vi "EuniceF_Project5.vi"() -> ()   [LabVIEW 2025]
panel:
  out "TemperatureChart":dbl(graph)
  out "RTD":dbl(slide) scale=100.0..110.0
  out "Vp,mV":dbl(slide) scale=0.0..100.0
  out "Vdiff,mV":dbl(slide) scale=0.0..100.0
  out "COLD":bool
  in  "STOP":bool
  out "HOT":bool
  out "Thermometer":dbl(slide) scale=0.0..100.0
  out "Vscc,V":dbl(slide) scale=-10.0..10.0
  out "AtoD":i16
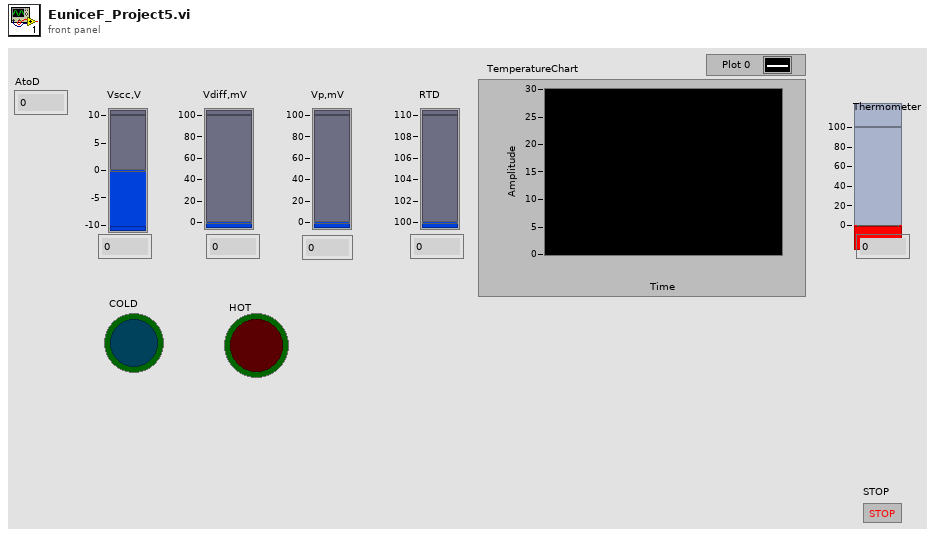
[diagram p1: front panel]
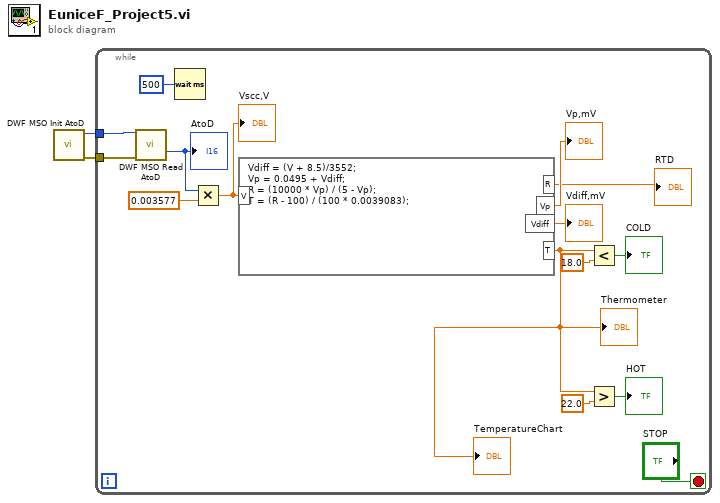
[diagram p0: block diagram]
diagram:
  n1 = call "DWF MSO Init AtoD.vi"() -> ("Error Out"=w1:errorcluster, "Instrument Handle Out"=w2:i32)  [unwired: 10 in]
  n2 = while {
    tunnel: w2 -> [w17]
    tunnel: w1 -> [w16]
    stop <- "STOP" stop-if-true
    n3 = call "DWF MSO Read AtoD.vi"("Instrument Handle In AtoD"=w17, "Error In"=w16) -> ("AtoD"=w15:i16)  [unwired: 12 in, 1 out]
    "AtoD" <- w15
    n4 = Wait (ms)(milliseconds to wait=u32 500) -> ()  [unwired: 1 out]
    n5 = Multiply(x=w15, y=0.003577) -> (x*y=w13:dbl)
    "Vscc,V" <- w13
    n6 = formula code="Vdiff = (V + 8.5)/3552;\nVp = 0.0495 + Vdiff;\nR = (10000 * Vp) / (5 - Vp);\nT = (R - 100) / (100 * 0.0039083);"("V"=w13) -> ("T"=w3:dbl, "Vdiff"=→"Vdiff,mV":dbl, "Vp"=→"Vp,mV":dbl, "R"=→"RTD":dbl)
    "Thermometer" <- w3
    "TemperatureChart" <- w3
    n7 = Less?(x=w3, y=18.0) -> (x < y?=→"COLD":bool)
    n8 = Greater?(x=w3, y=22.0) -> (0:→"HOT":bool)
  }
